vi "Get Version.vi"(8 "error in (no error)":errorcluster, 11 "VI Reference in":refnum<vi>) -> (0 "error out":errorcluster, 2 "Version":T1, 3 "VI Reference out":refnum<vi>)   [LabVIEW 2021, in "CIFCoreCommon.lvlib"]
uses:
  CIFCoreCommon.lvlib
  Typedef/Version.ctl
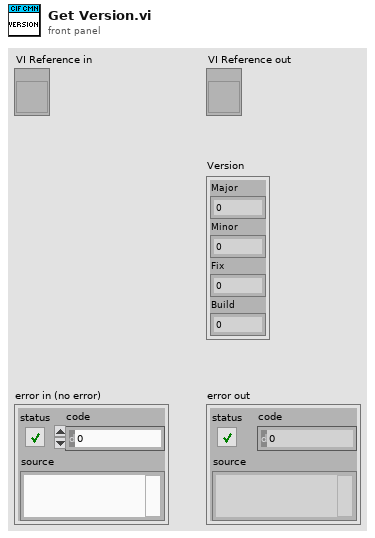
[diagram p1: front panel]
types:
  T1 = typedef "CIFCoreCommon.lvlib/Version.ctl" = cluster{"Major":i32, "Minor":i32, "Fix":i32, "Build":i32}
  T2 = cluster{"Major":u16, "Minor":u16, "Fix":u16, "Build":u16}
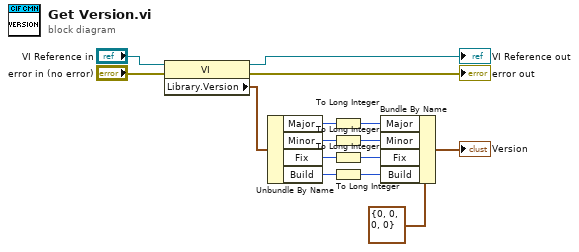
[diagram p0: block diagram]
diagram:
  n1 = property class="VI"(reference="VI Reference in", error in="error in (no error)") -> (reference out=→"VI Reference out":refnum<vi>, error out=→"error out":errorcluster, "Library.Version"=w13:T2)
  n2 = Unbundle By Name(w13) -> ("Major"=w10:u16, "Minor"=w3:u16, "Fix"=w6:u16, "Build"=w7:u16)
  n3 = To Long Integer(number=w10) -> (32bit integer=w9:i32)
  n4 = To Long Integer(number=w3) -> (32bit integer=w4:i32)
  n5 = To Long Integer(number=w6) -> (32bit integer=w5:i32)
  n6 = To Long Integer(number=w7) -> (32bit integer=w8:i32)
  n7 = Bundle By Name(cluster=T1 {"Major"=0, "Minor"=0, "Fix"=0, "Build"=0} ("Version 2"), "Major"=w9, "Minor"=w4, "Fix"=w5, "Build"=w8) -> (→"Version":T1)
